vi "updateWeekDay.vi"(11 "Cron in":T1) -> (3 "Cron Time":T1)   [LabVIEW 2013, in "openCron.lvlib" / "Cron.lvclass"]
uses:
  Cron.lvclass
  CronTime -- cluster.ctl
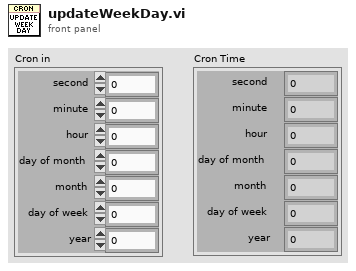
[diagram p1: front panel]
types:
  T1 = typedef "openCron.lvlib/Cron.lvclass/CronTime -- cluster.ctl" = cluster{"second":i32, "minute":i32, "hour":i32, "day of month":i32, "month":i32, "day of week":i32, "year":i32}
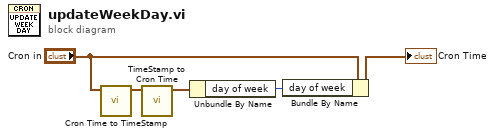
[diagram p0: block diagram]
diagram:
  n1 = call "Cron Time to TimeStamp.vi"("Cron Time"="Cron in") -> ("Time Stamp"=w5:timestamp)  [unwired: 10 in]
  n2 = call "TimeStamp to Cron Time.vi"("Time Stamp"=w5) -> ("Cron Time"=w2:T1)  [unwired: 10 in]
  n3 = Unbundle By Name(w2) -> ("day of week"=w1:i32)
  n4 = Bundle By Name(cluster="Cron in", "day of week"=w1) -> (→"Cron Time":T1)
